vi "Main_Window.vi"() -> ()   [LabVIEW 2017]
panel:
  out "Connection 6":bool
  out "Connection 5":bool
  out "Connection 4":bool
  out "Connection 3":bool
  out "Connection 2":bool
  out "Connection 1":bool
  in  "Data Collection":bool
  in  "Equipment Calibration":bool
  # "AIARG Sidewall Balance Driver"
  # "Welcome To AIARG Sidewall Balance Driver!\nPlease select an option below:"
  # "This option allows the user to calibrate the equipment."
  # "IT IS RECOMMENDED TO CALIBRATE THE EQUIPMENT BEFORE USE!"
  # "This option allows the user to collect data."
  # "I/O Connection Status"
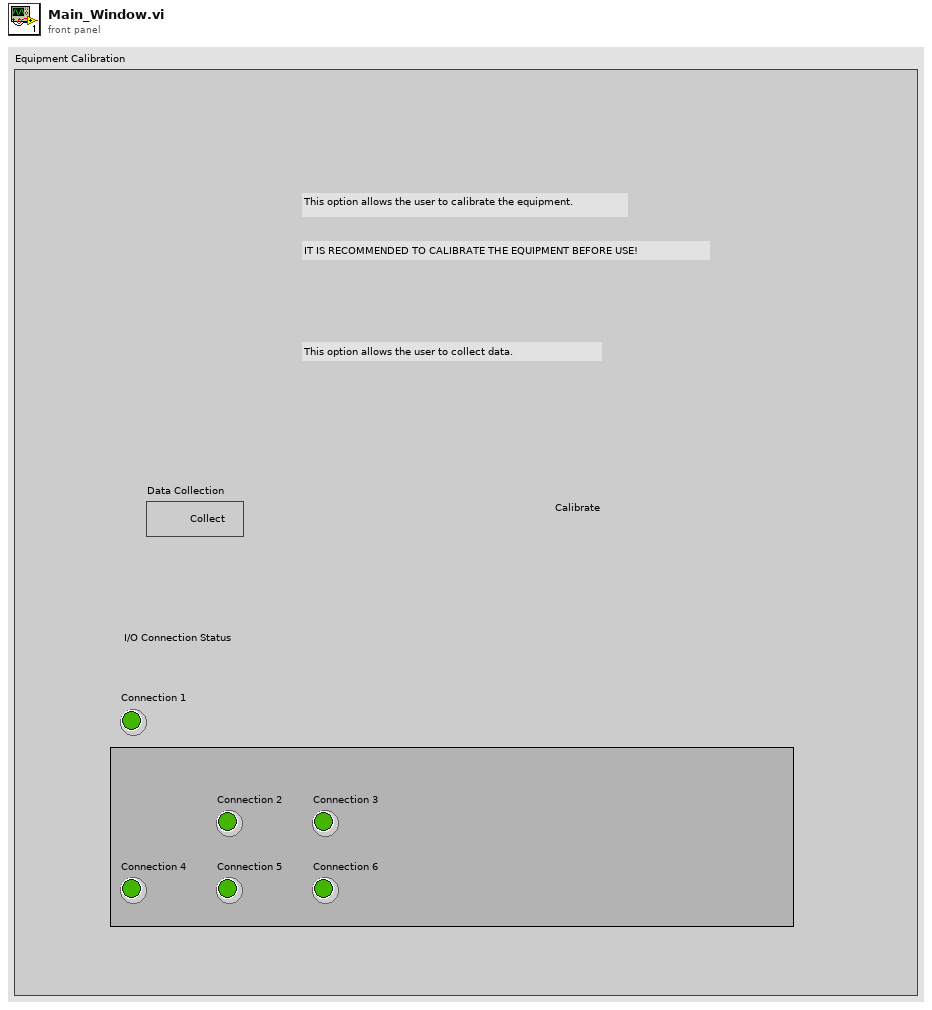
[diagram p1: front panel]
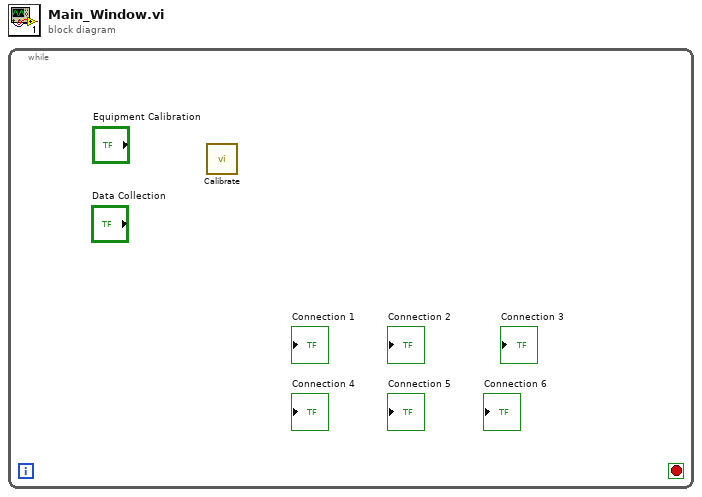
[diagram p0: block diagram]
diagram:
  n1 = while {
    stop <- _ stop-if-true
    n2 = call "Calibrate.vi"() -> ()  [unwired: 12 in]
  }
